vi "ReadABF.vi"(4 "에러 입력":errorcluster, 6 "FilePath":path=path "C:/Users/KimYG/Experimental Data/Flocculus_Ex vivo/6. Plsticity/190119/190119_#07/190119__0026.abf", 7 "ABFFIO.lvclass IN":refnum<class "ABFFIO.lvclass">) -> (0 "error out":errorcluster caption="에러 출력", 3 "ABFFIO.lvclass OUT":refnum<class "ABFFIO.lvclass">)   [LabVIEW 2017, in "ABFFIO.lvclass"]
uses:
  ABFFIO.lvclass
  ABFFIO.lvclass/ABFFIO.ctl
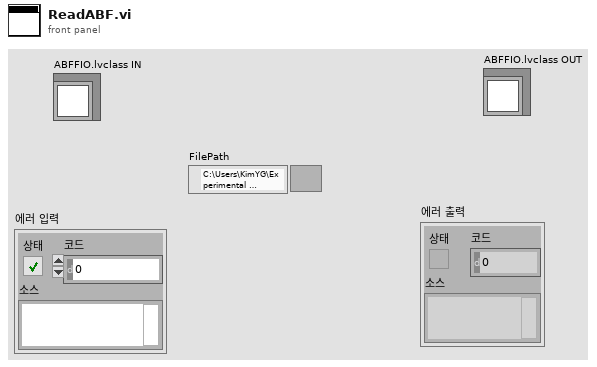
[diagram p1: front panel]
types:
  T1 = enum16{"big-endian, network order", "native, host order", "little-endian"}
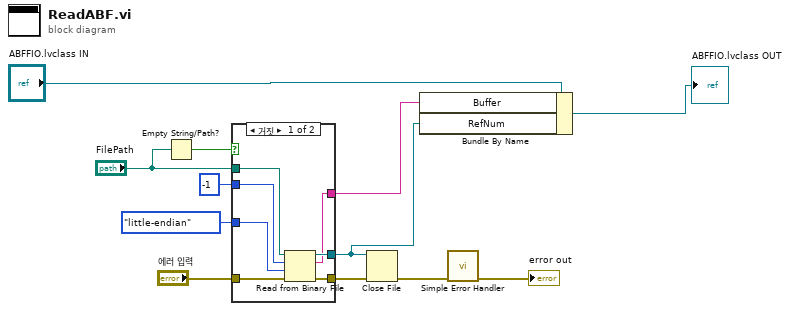
[diagram p0: block diagram]
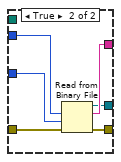
[diagram p2: hidden frame]
diagram:
  n1 = Empty String/Path?(string/path="FilePath") -> (empty?=w5:bool)
  n2 = case shown="거짓" w5 {
    tunnel: T1."little-endian" ("바이트 순서(0:big-endian, network order)") -> [w19 w23]
    tunnel: [w18 w20] -> w2
    tunnel: [w17 w24] -> w11
    tunnel: "에러 입력" -> [w16 w25]
    tunnel: -1 ("numBytes") -> [w15 w22]
    tunnel: [w14 w21] -> w3
    tunnel: "FilePath" -> [w13 _]
    frame False {
      n3 = Read from Binary File(8:w16, 9:w19, 10:w15, 11:w13) -> (0:w17:errorcluster, 2:w14:string, 3:w18:refnum<file>)  [unwired: 2 in, 1 out]
    }
    frame True {
      n4 = Read from Binary File(8:w25, 9:w23, 10:w22) -> (0:w24:errorcluster, 2:w21:string, 3:w20:refnum<file>)  [unwired: 3 in, 1 out]
    }
  }
  n5 = Close File(refnum=w2, error in=w11) -> (error out=w10:errorcluster)  [unwired: 1 out]
  n6 = Bundle By Name(cluster="ABFFIO.lvclass IN", "Buffer"=w3, "RefNum"=w2) -> (→"ABFFIO.lvclass OUT":refnum<class "ABFFIO.lvclass">)
  n7 = call <vilib>:"Simple Error Handler.vi"("error in (no error)"=w10) -> ("error out"=→"error out":errorcluster)  [unwired: 4 in, 4 out]
